vi "Write ROI.vi"(8 "error in (no error)":errorcluster, 10 "ROI":T1, 11 "ROI Name Dialog in":refnum<class "ROI Name Dialog.lvclass">) -> (0 "error out":errorcluster, 3 "ROI Name Dialog out":refnum<class "ROI Name Dialog.lvclass">)   [LabVIEW 2014, in "ROI Name Dialog.lvlib" / "ROI Name Dialog.lvclass"]
uses:
  ROI Name Dialog.lvclass
  ROI Name Dialog.lvclass/ROI Name Dialog.ctl
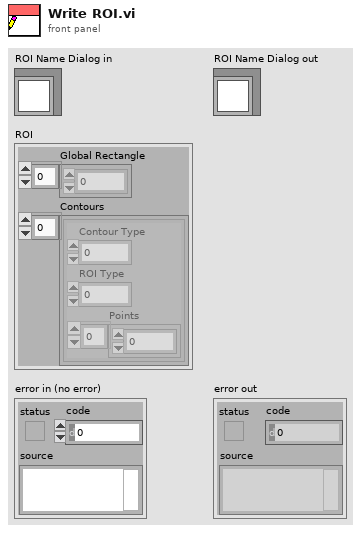
[diagram p1: front panel]
types:
  T1 = cluster{"Global Rectangle":i32[], "Contours":cluster{"Contour Type":u32, "ROI Type":u32, "Points":i32[]}[]}
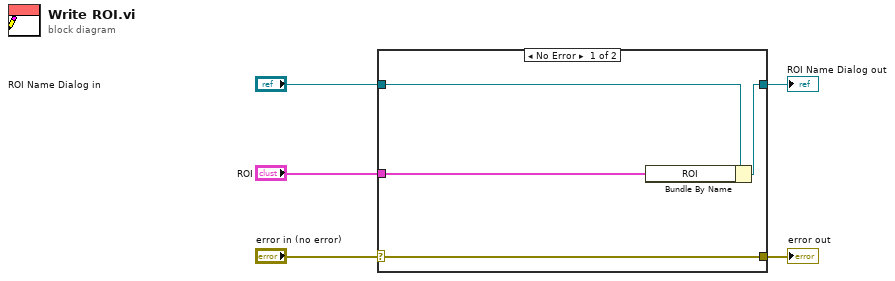
[diagram p0: block diagram]
diagram:
  n1 = case shown="No Error" "error in (no error)" {
    selector: "error in (no error)" -> [w9 w10]
    tunnel: [w9 w10] -> w4
    tunnel: [w7 w11] -> w2
    tunnel: "ROI Name Dialog in" -> [w8 w11]
    tunnel: "ROI" -> [w6 _]
    frame No Error {
      n2 = Bundle By Name(cluster=w8, "ROI"=w6) -> (w7:refnum<class "ROI Name Dialog.lvclass">)
    }
    frame Error {
    }
  }
  "error out" <- w4
  "ROI Name Dialog out" <- w2
